vi "Format Path and Filename.vi"(6 "append? (F)":bool, 8 "error in":errorcluster, 9 "Type (TDMS)":T1, 10 "filename":string, 11 "path":path) -> (0 "error out":errorcluster, 2 "filename without extension":string, 3 "path":path)   [LabVIEW 2016, in "LV to ITX.lvclass"]
uses:
  LV to ITX.lvclass
  Typedefs/Filetype--enum.ctl
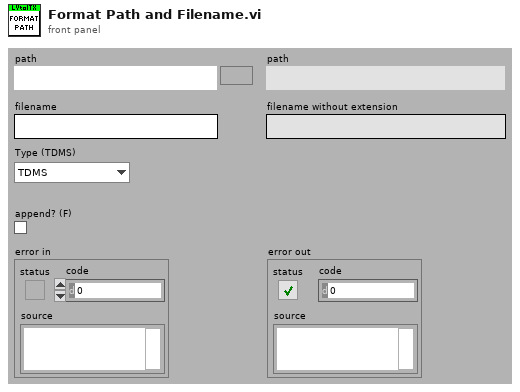
[diagram p1: front panel]
types:
  T1 = typedef "LV to ITX.lvclass/Filetype--enum.ctl" = enum16{"TDMS", "ITX", "DAT"}
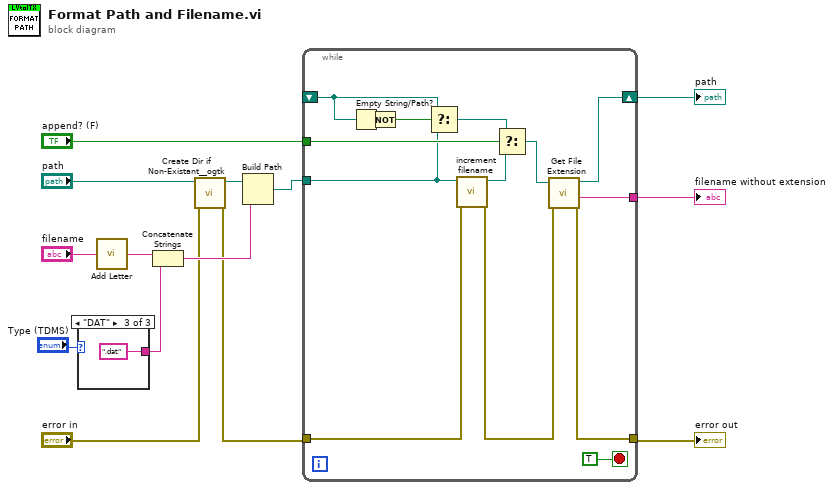
[diagram p0: block diagram]
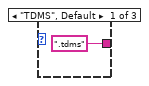
[diagram p2: hidden frame]
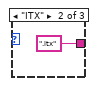
[diagram p3: hidden frame]
diagram:
  n1 = case shown="\"DAT\"" "Type (TDMS)" {
    tunnel: [".tdms" ("string") ".itx" ("string") ".dat" ("string")] -> w1
    frame "TDMS", Default {
    }
    frame "ITX" {
    }
    frame "DAT" {
    }
  }
  n2 = call "Add Letter.vi"("String"="filename") -> ("output string"=w12:string)
  n3 = Concatenate Strings(w12, w1) -> (w14:string)
  n4 = call <userlib>:"Create Dir if Non-Existant__ogtk.vi"("error in (no error)"="error in", "Directory Path"="path") -> ("error out"=w4:errorcluster, "dup Directory Path"=w6:path)  [unwired: 7 in, 1 out]
  n5 = Build Path(base path=w6, name or relative path=w14) -> (appended path=w3:path)
  n6 = while {
    tunnel: [w31] -> w11
    tunnel: "append? (F)" -> [w29]
    tunnel: w3 -> [w22]
    shift-right: [w20] -> w9
    shift-left: _ -> [w26]
    tunnel: w4 -> [w19]
    tunnel: [w24] -> w8
    stop <- TRUE stop-if-true
    n7 = Empty String/Path?(string/path=w26) -> (empty?=w28:bool)
    n8 = Not(x=w28) -> (.not. x?=w27:bool)
    n9 = Select(t=w26, s=w27, f=w22) -> (s? t:f=w25:path)
    n10 = call <userlib>:"increment filename.vi"("error in (no error)"=w19, "path"=w22) -> ("error out"=w18:errorcluster, "modified path"=w23:path)  [unwired: 8 in]
    n11 = Select(t=w25, s=w29, f=w23) -> (s? t:f=w21:path)
    n12 = call <vilib>:"Get File Extension.vi"("error in (no error)"=w18, "file"=w21) -> ("error out"=w24:errorcluster, "filename without extension"=w31:string, "dup file"=w20:path)  [unwired: 7 out]
  }
  "filename without extension" <- w11
  "path" <- w9
  "error out" <- w8
